vi "QCPFileRead.vi"(9 "Path Relative?":bool=TRUE, 10 "File Path":string, 11 "QCP Data Block In":T1) -> (0 "error out":errorcluster, 3 "QCP Data Block Out":T1)   [LabVIEW 2015]
uses:
  <userlib>/836-Library/System/QCP_Support_Code/QCP_Data_Block.ctl
  <vilib>/Utility/error.llb/Error Cluster From Error Code.vi
  <vilib>/Utility/file.llb/Read From Spreadsheet File (string).vi
  <vilib>/ErrorRing/Error Ring.xnode
panel:
  out "appended path":path
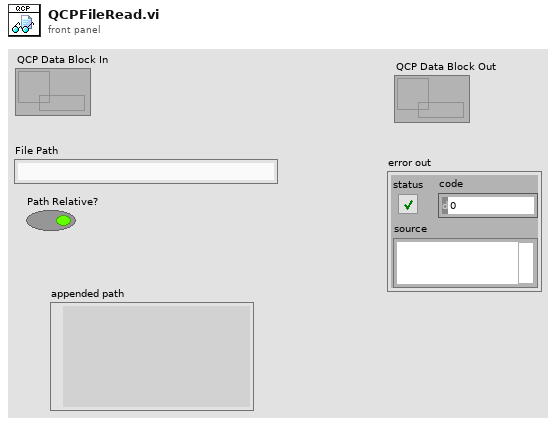
[diagram p1: front panel]
types:
  T1 = typedef "QCP_Data_Block.ctl" = refnum<data-value>
  T2 = cluster{"all rows":string[], "all rows":string[]}
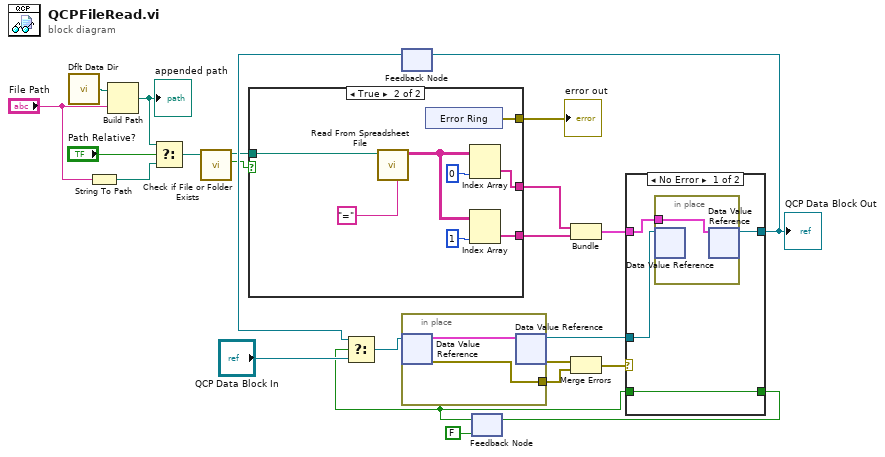
[diagram p0: block diagram]
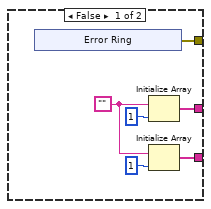
[diagram p2: hidden frame]
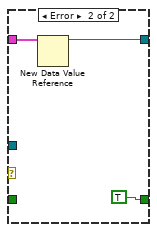
[diagram p3: hidden frame]
diagram:
  n1 = call <vilib>:"Dflt Data Dir.vi"() -> ("App:Default Data Directory"=w1:path)
  n2 = String To Path(string="File Path") -> (path=w3:path)
  n3 = Build Path(base path=w1, name or relative path="File Path") -> (appended path=w2:path)
  "appended path" <- w2
  n4 = Select(t=w2, s="Path Relative?", f=w3) -> (s? t:f=w5:path)
  n5 = call <vilib>:"Check if File or Folder Exists.vi"("path"=w5) -> ("file or folder exists?"=w7:bool, "dup path"=w8:path)  [unwired: 8 in, 1 out]
  n6 = case shown="True" w7 {
    tunnel: [w24 w38] -> w12
    tunnel: [w25 w37] -> w11
    tunnel: w8 -> [_ w36]
    tunnel: [w29 w35] -> w6
    frame False {
      w26 = ""
      n7 = xnode "Error Ring"() -> ("error out"=w29:errorcluster)
      n8 = Initialize Array(w26, 1 ("dimension size")) -> (w24:string[])
      n9 = Initialize Array(w26, 1 ("dimension size")) -> (w25:string[])
    }
    frame True {
      n10 = call-poly <vilib>:"Read From Spreadsheet File.vi"("delimiter (\\t)"="=" ("delimiter (\\t)"), "file path (dialog if empty)"=w36) -> ("all rows"=w40:string[][])  [unwired: 5 in, 4 out]
      n11 = xnode "Error Ring"() -> ("error out"=w35:errorcluster)
      n12 = Index Array(array=w40, index (col)=0 ("disabled index (col)")) -> (element=w38:string[])  [unwired: 1 in]
      n13 = Index Array(array=w40, index (col)=1 ("disabled index (col)")) -> (element=w37:string[])  [unwired: 1 in]
    }
  }
  "error out" <- w6
  n14 = feedback #1() -> (w13:T1)  [unwired: 1 in]
  n15 = feedback #2(FALSE) -> (w14:bool)
  n16 = Select(t=w13, s=w14, f="QCP Data Block In") -> (s? t:f=w15:T1)
  n17 = in-place {
    in-place-border: [w44] -> w22
    n18 = in-place-dvr #3(w15) -> (w45:cluster{string[], string[]}, w44:errorcluster)
    n19 = in-place-dvr #3(w45) -> (w20:T1, w23:errorcluster)
  }
  n20 = Bundle("all rows"=w12, "all rows"=w11) -> (w10:T2)  [unwired: 1 in]
  n21 = Merge Errors(w23, w22) -> (w21:errorcluster)
  n22 = case shown="No Error" w21 {
    tunnel: [w49 w51] -> w19
    tunnel: w20 -> [w48 _]
    tunnel: [w47 TRUE] -> w18
    tunnel: w14 -> [w47 _]
    tunnel: w10 -> [w46 w52]
    frame No Error {
      n23 = in-place {
        in-place-border: w46 -> [w50]
        n24 = in-place-dvr #4(w48) -> ()  [unwired: 2 out]
        n25 = in-place-dvr #4(w50) -> (w49:T1)  [unwired: 1 out]
      }
    }
    frame Error {
      n26 = New Data Value Reference(data value=w52) -> (data value reference=w51:refnum<data-value>)  [unwired: 1 in, 1 out]
    }
  }
  "QCP Data Block Out" <- w19
  n27 = feedback-in #1(w19) -> ()
  n28 = feedback-in #2(w18) -> ()
